vi "Read UI Display.vi"(0 "GEA2 Reference In":refnum<k24>, 11 "Error In":errorcluster) -> (4 "GEA2 Reference Out":refnum<k24>, 6 "Justice League UI":T2, 8 "Justice League SB":T1, 13 "LED's Out 0-79":bool[](array[boolean]), 14 "Convert raw data":string[](array[string]), 15 "Error Out":errorcluster)   [LabVIEW 2016]
doc: "This VI is used to verify the display on the HEUI."
uses:
  Q:/Common/DLLs/GEA3/GeaCommunication.dll
  Common/DLLs/GEA3/GeaCommunication.dll
  type defs/UI_LEDs.ctl
  type defs/SB_LEDs.ctl
  Common/LabVIEW GEA2 Toolkit/LabVIEW_GEA2_Toolkit.lvlibp/type defs/ERD Read Data In.ctl
  Common/LabVIEW GEA2 Toolkit/LabVIEW_GEA2_Toolkit.lvlibp/type defs/Data Type.ctl
  Common/LabVIEW GEA2 Toolkit/LabVIEW_GEA2_Toolkit.lvlibp/type defs/Source_Destination.ctl
  Common/LabVIEW GEA2 Toolkit/LabVIEW_GEA2_Toolkit.lvlibp
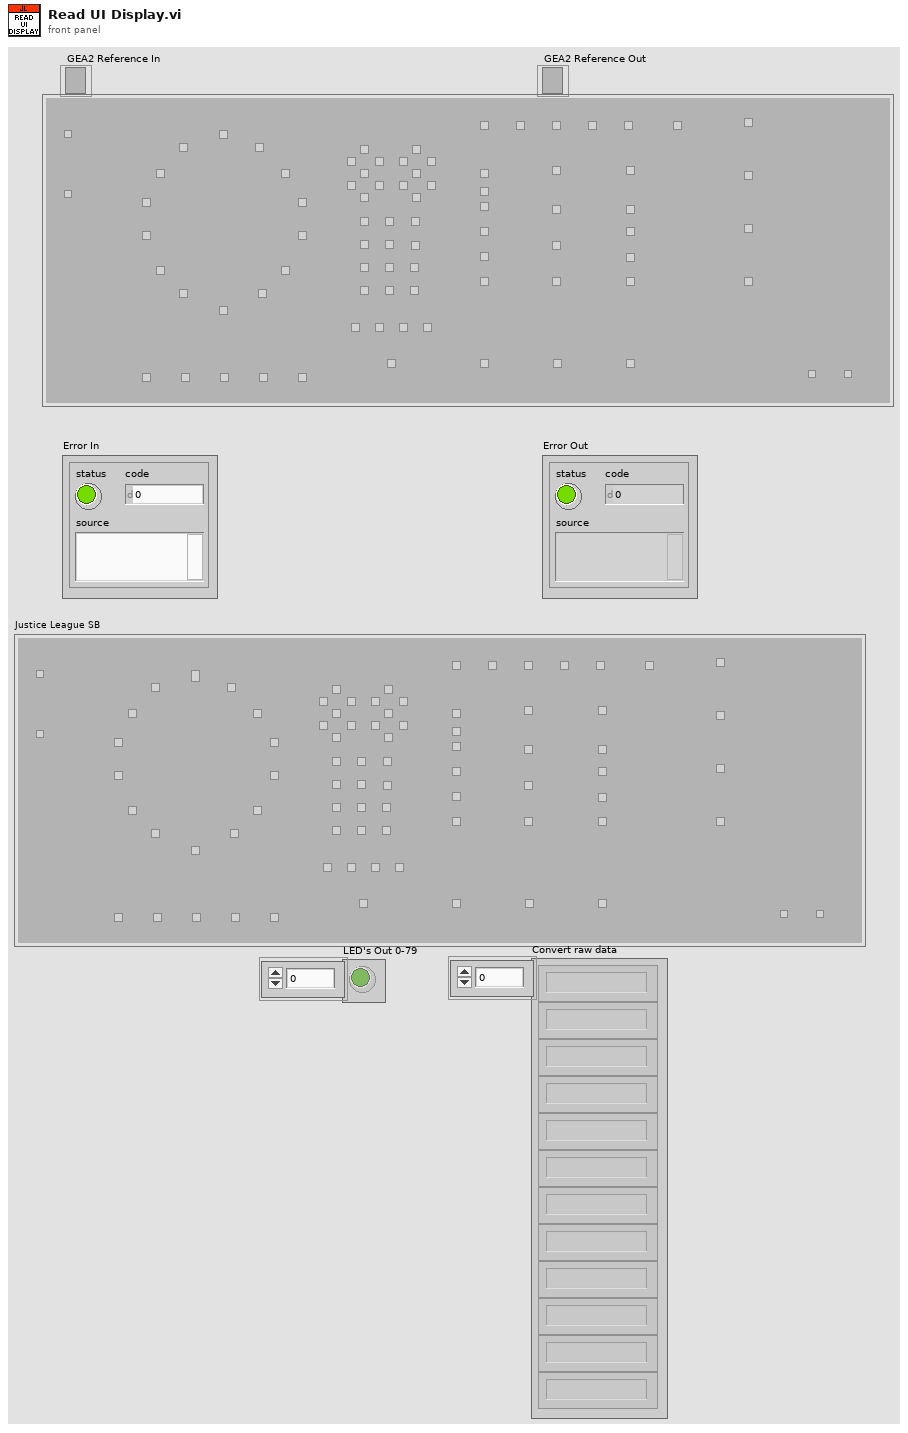
[diagram p1: front panel]
types:
  T1 = typedef "SB_LEDs.ctl" = cluster{"Z101 - Start/Pause":bool, "Z - unpop?":bool, "Z103 - Encoder 0":bool, "Z104 - Encoder 13":bool, "Z105 - Encoder 12":bool, "Z106 - Encoder 11":bool, "Z107 - Encoder 10":bool, "Z108 - Encoder 09":bool, "Z109 - Encoder 08":bool, "Z110 - Encoder 07":bool, "Z111 - Encoder 06":bool, "Z112 - Encoder 05":bool, "Z113 - Encoder 04":bool, "Z114 - Encoder 03":bool, "Z115 - Encoder 02":bool, "Z116 - Encoder 01":bool, "Z117 - Bar 1":bool, "Z118 - Bar 2":bool, "Z119 - Bar 3":bool, "Z120 - Bar 4":bool, "Z121 - Bar 5":bool, "Z122 - SSD1:A":bool, "Z123 - SSD1:B":bool, "Z124 - SSD1:C":bool, "Z125 - SSD1:D":bool, "Z126 - SSD1:E":bool, "Z127 - SSD1:F":bool, "Z128 - SSD1:G":bool, "Z129 - SSD2:A":bool, "Z130 - SSD2:B":bool, "Z131 - SSD2:C":bool, "Z132 - SSD2:D":bool, "Z133 - SSD2:E":bool, "Z134 - SSD2:F":bool, "Z135 - SSD2:G":bool, "Z136 - Pause 2":bool, "Z137 - Pause 3":bool, "Z138 - Control Lock 1":bool, "Z139 - Control Lock 2":bool, "Z140 - Control Lock 3":bool, "Z142 - Sensing 1":bool, "Z142 -Sensing 2":bool, "Z143 - Sensing 3":bool, "Z144 - Extra Status 1":bool, "Z145 - Extra Status 2":bool, "Z146 - Extra Status 3":bool, "Z147 - Extra Status 4":bool, "Z148 - Status 1":bool, "Z149 - Status 2":bool, "Z150 - Status 3":bool, "Z151 - Status 4":bool, "Z152 - Status 5":bool, "Z153 - Status 6":bool, "Z154 - Default Time 5":bool, "Z155 - Default Time 4":bool, "Z153 - Default Time 3":bool, "Z157 -Default Time 2":bool, "Z158 - Default Time 1":bool, "Z159 - Default Time 0":bool, "Z160 - More Dry":bool, "Z161 - Dry":bool, "Z162 - Less Dry":bool, "Z163 - Damp":bool, "Z164 - High":bool, "Z165 - Medium":bool, "Z166 - Extra Low":bool, "Z167 - No Heat":bool, "Z168 - Volume":bool, "Z169 - Damp Alert":bool, "Z170 - Extended Tumble":bool, "Z171 - Time Decrement":bool, "Z172 - Time Increment":bool, "Z173 - eDry":bool, "Z174 -My Cycle":bool, "Z175 - Delay Dry":bool, "Z176 - Clean Lint Filter 1":bool, "Z177 - Clean Lint Filter 2":bool, "Z178 - Clean Lint Filter 3":bool, "Z179 - Pause 1":bool, "OFF - OFF":bool, "MAX - MAX":bool, "Z165B -Low":bool}
  T2 = typedef "UI_LEDs.ctl" = cluster{"Z301 - Encoder 0":bool, "Z302 - Encoder 13":bool, "Z303 - Encoder 12":bool, "Z304 - Encoder 11":bool, "Z305 - Encoder 10":bool, "Z306 - Encoder 09":bool, "Z307 - Encoder 08":bool, "Z308 - Encoder 07":bool, "Z309 - Encoder 06":bool, "Z310 - Encoder 05":bool, "Z311 - Encoder 04":bool, "Z312 - Encoder 03":bool, "Z313 - Encoder 02":bool, "Z314 - Encoder 01":bool, "Z315 - Unpopulated":bool, "Z316 - Unpopulated":bool, "Z317 - SSD1:A":bool, "Z318 - SSD1:B":bool, "Z319 - SSD1:G":bool, "Z320 - SSD1:C":bool, "Z321 - SSD1:D":bool, "Z322 - SSD1:E":bool, "Z323 - SSD1:F":bool, "Z324 - Pause 1":bool, "Z325 - Control Lock 1":bool, "Z326 - Sensing 1":bool, "Z327 - Clean Lint Filter 1":bool, "Z328 - Extra Status 1":bool, "Z329 - Extra Status 2":bool, "Z330 - Clean Lint Filter 2":bool, "Z331 -Sensing 2":bool, "Z332 - Unpopulated":bool, "Z333 - SSD2:A":bool, "Z334 - SSD2:B":bool, "Z335 - SSD2:G":bool, "Z345 - SSD2:C":bool, "Z336 - SSD2:D":bool, "Z337 - SSD2:E":bool, "Z338 - SSD2:F":bool, "Z339 - Pause 3":bool, "Z340 - Control Lock 3":bool, "Z353 - Sensing 3":bool, "Z342 - Clean Lint Filter 3":bool, "Z344 - Extra Status 3":bool, "Z346 - Extra Status 4":bool, "Z341 - Pause 2":bool, "Z343 - Control Lock 2":bool, "Z347 - Unpopulated":bool, "Z348 -My Cycle":bool, "Z349 - Delay Dry":bool, "Z350 - Volume":bool, "Z351 - Damp Alert":bool, "Z352 - Bar 1":bool, "Z354 - Bar 2":bool, "Z355 - Bar 3":bool, "Z356 - Bar 4":bool, "Z357 - Bar 5":bool, "Z358 - eDry":bool, "Z359 - Time Increment":bool, "Z360 - Time Decrement":bool, "Z361 - Extended Tumble":bool, "Z362 - Unpopulated":bool, "Z363 - Unpopulated":bool, "Z364 - Unpopulated":bool, "Z365 - Status 1":bool, "Z366 - Status 3":bool, "Z367 - Default Time 5":bool, "Z368 - Default Time 4":bool, "Z369 - Default Time 3":bool, "Z370 - Dry":bool, "Z371 - Status 2":bool, "Z372 -Default Time 2":bool, "Z373 - Default Time 1":bool, "Z374 - Unpopulated":bool, "Z375 - Default Time 0":bool, "Z376 - No Heat":bool, "Z377 - Unpopulated":bool, "Z378 - Unpopulated":bool, "Z379 - Unpopulated":bool, "Z380 - Unpopulated":bool, "Z381 - Status 4":bool, "Z382 - Status 6":bool, "Z383 - More Dry":bool, "Z384 - High":bool, "Z385 - Medium":bool, "Z386 -Low":bool, "Z387 - Status 5":bool, "Z388 - Less Dry":bool, "Z388 - Extra Low":bool, "Z390 - Unpopulated":bool, "Z391 - Damp":bool, "Z392 - Unpopulated":bool, "Z393 - Unpopulated":bool, "Z394 - Unpopulated":bool, "Z395 - Unpopulated":bool, "Z396 - Unpopulated":bool, "Z101 - unpop?":bool, "Z102 - Start/Pause":bool, "OFF - OFF":bool, "MAX - MAX":bool}
  T3 = typedef "LabVIEW_GEA2_Toolkit.lvlibp/Source_Destination.ctl" = cluster{"Source":u8, "Destination":u8}
  T4 = typedef "LabVIEW_GEA2_Toolkit.lvlibp/ERD Read Data In.ctl" = cluster{"ERD Number":u16, "Data Type":T5}
  T5 = typedef "LabVIEW_GEA2_Toolkit.lvlibp/Data Type.ctl" = enum16{"string", "boolean", "uint8_t", "uint16_t", "uint32_t", "uint64_t", "int8_t", "int16_t", "int32_t", "int64_t"}
  T6 = typedef "LabVIEW_GEA2_Toolkit.lvlibp/ERD Read Data Out.ctl" = cluster{"ERD Number":u16, "Data":string}
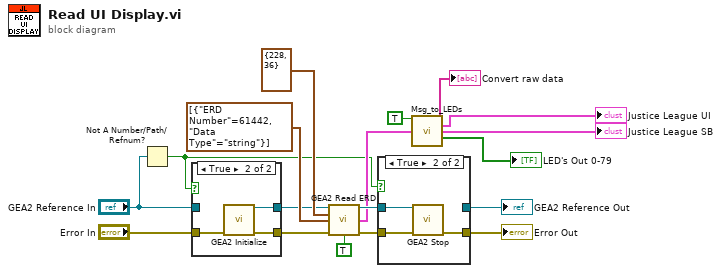
[diagram p0: block diagram]
diagram:
  n1 = Not A Number/Path/Refnum?(number/path/refnum="GEA2 Reference In") -> (NaN/Path/Refnum?=w6:bool)
  n2 = case shown="True" w6 {
    tunnel: [w19 w23] -> w14
    tunnel: "Error In" -> [w19 w22]
    tunnel: [w20 w21] -> w12
    tunnel: "GEA2 Reference In" -> [w20 _]
    frame False {
    }
    frame True {
      n3 = call "GEA2 Initialize.vi"("error in"=w22) -> ("GEA2 Reference Out"=w21:refnum<k24>, "error out"=w23:errorcluster)  [unwired: 12 in, 1 out]
    }
  }
  n4 = call "GEA2 Read ERD.vi"("GEA2 Reference In"=w12, "GEA Inputs"=T3 {"Source"=228, "Destination"=36}, "Read ERD List"=T4[] [{"ERD Number"=61442, "Data Type"=enum."string"}], "Error In"=w14, "Verify ERD Response?"=TRUE) -> ("GEA2 Reference Out"=w10:refnum<k24>, "ERD Data Out"=w8:T6[], "Error Out"=w15:errorcluster)  [unwired: 7 in, 1 out]
  n5 = case shown="True" w6 {
    tunnel: w15 -> [w24 w28]
    tunnel: [w24 w27] -> w9
    tunnel: [w25 _] -> w11
    tunnel: w10 -> [w25 w26]
    frame False {
    }
    frame True {
      n6 = call "GEA2 Stop.vi"("GEA2 Reference In"=w26, "Error In"=w28) -> ("Error Out"=w27:errorcluster)  [unwired: 13 in]
    }
  }
  "GEA2 Reference Out" <- w11
  "Error Out" <- w9
  n7 = call "Msg_to_LEDs.vi"("SingleBoard?"=TRUE, "ERD Data Out"=w8) -> ("Convert raw data"=→"Convert raw data":string[], "Justice League UI"=→"Justice League UI":T2, "Justice League SB"=→"Justice League SB":T1, "LED's Out 0-79"=→"LED's Out 0-79":bool[])  [unwired: 10 in]
